vi "TEST_COMMANDS.vi"() -> ()   [LabVIEW 2020]
panel:
  out "?":bool
  in  "ENTER COMMANDS":string
  out "OUT":string
  in  "VISA resource name":refnum<visa-resource-name>
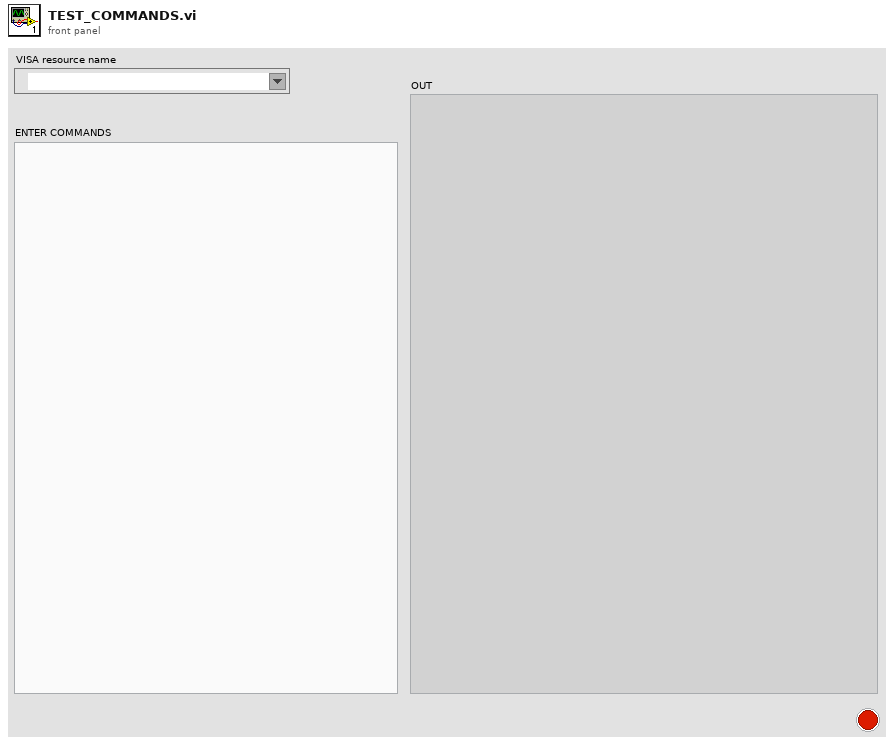
[diagram p1: front panel]
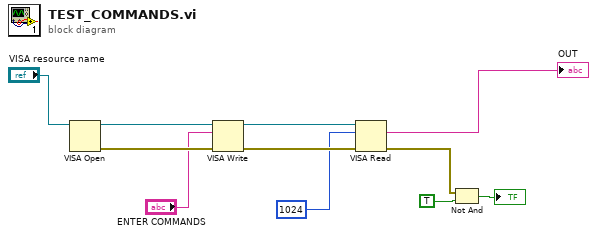
[diagram p0: block diagram]
diagram:
  n1 = VISA Open(VISA resource name="VISA resource name") -> (VISA resource name=w11:refnum<visa-resource-name>, error out=w9:errorcluster)  [unwired: 4 in]
  n2 = VISA Write(VISA resource name=w11, write buffer="ENTER COMMANDS", error in (no error)=w9) -> (VISA resource name out=w10:refnum<visa-resource-name>, error out=w8:errorcluster)  [unwired: 1 out]
  n3 = VISA Read(VISA resource name=w10, byte count=u32 1024, error in (no error)=w8) -> (read buffer=→"OUT":string, error out=w1:errorcluster)  [unwired: 2 out]
  n4 = Not And(1:TRUE ("y"), 2:w1) -> (0:→"?":bool)
